vi "NATS PUB.vi"(6 "timeout ms (conn default)":i32=-2, 7 "reply-to":string, 8 "error in":errorcluster, 9 "payload":string, 10 "subject":string, 11 "nats connection in":T1={"connection ID"=refnum, "server INFO"="", "timeout ms"=5000, "verbose?"=FALSE, "server headers?"=FALSE, "client headers?"=FALSE}) -> (0 "error out":errorcluster, 3 "dup nats connection":T1={"connection ID"=refnum, "server INFO"="", "timeout ms"=5000, "verbose?"=FALSE, "server headers?"=FALSE, "client headers?"=FALSE})   [LabVIEW 2013, in "NATS Core.lvlib"]
doc: "Publishes a message to the NATS server."
uses:
  NATS Core.lvlib
  Controls/nats connection.ctl
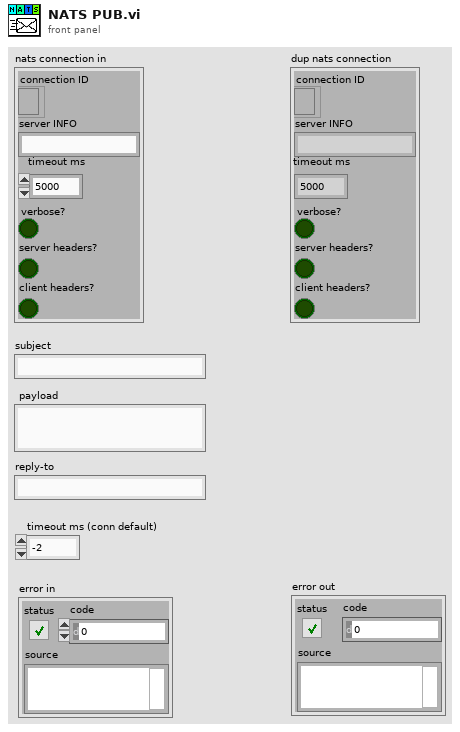
[diagram p1: front panel]
types:
  T1 = typedef "NATS Core.lvlib/nats connection.ctl" = cluster{"connection ID":refnum<k5>, "server INFO":string, "timeout ms":i32, "verbose?":bool, "server headers?":bool, "client headers?":bool}
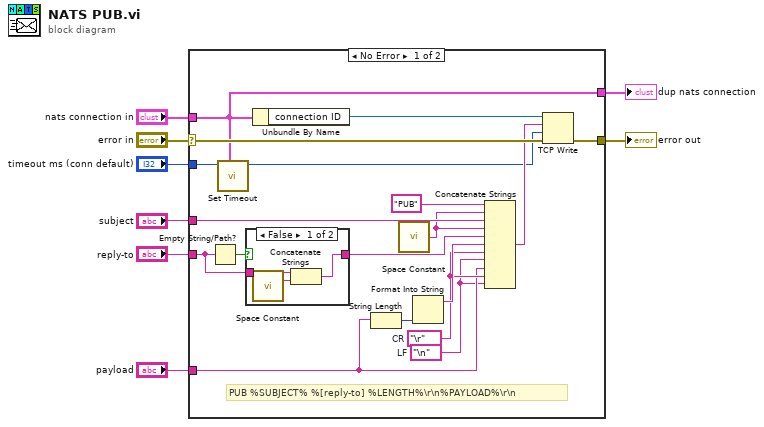
[diagram p0: block diagram]
diagram:
  n1 = case shown="No Error" "error in" {
    selector: "error in" -> [w26 w32]
    tunnel: "nats connection in" -> [w18 w31]
    tunnel: "timeout ms (conn default)" -> [w17 _]
    tunnel: [w24 w32] -> w5
    tunnel: "subject" -> [w22 _]
    tunnel: "payload" -> [w10 _]
    tunnel: [w18 w31] -> w2
    tunnel: "reply-to" -> [w13 _]
    frame No Error {
      w9 = "\n"  # LF
      w11 = "\r"  # CR
      # "PUB %SUBJECT% %[reply-to] %LENGTH%\\r\\n%PAYLOAD%\\r\\n"
      n2 = Empty String/Path?(string/path=w13) -> (empty?=w14:bool)
      n3 = call "Set Timeout.vi"("nats connection in"=w18, "timeout ms in"=w17) -> ("timeout ms out"=w16:i32)  [unwired: 9 in]
      n4 = case shown="False" w14 {
        tunnel: w13 -> [w29 w30]
        tunnel: [w27 w30] -> w12
        frame False {
          n5 = call <vilib>:"Space Constant.vi"() -> ("String"=w28:string)
          n6 = Concatenate Strings(w29, w28) -> (w27:string)
        }
        frame True {
        }
      }
      n7 = Unbundle By Name(w18) -> ("connection ID"=w25:refnum<k5>)
      n8 = String Length(string=w10) -> (length=w20:i32)
      n9 = call <vilib>:"Space Constant.vi"() -> ("String"=w21:string)
      n10 = Format Into String(w20) -> (resulting string=w15:string)  [unwired: 3 in, 1 out]
      n11 = Concatenate Strings("PUB", w21, w22, w21, w12, w15, w11, w9, w10, w11, w9) -> (w19:string)
      n12 = TCP Write(connection ID=w25, data in=w19, error in (no error)=w26, 9:w16) -> (error out=w24:errorcluster)  [unwired: 2 out]
    }
    frame Error {
    }
  }
  "error out" <- w5
  "dup nats connection" <- w2
